vi "SR_J-Input Cycle.vi"(8 "error in (no error)":errorcluster, 10 "RDS Msg Q in":refnum<user-event>, 11 "Joystick":T1) -> (0 "error out":errorcluster, 2 "RDS Msg Q out":refnum<user-event>, 3 "Joystick Out":T1)   [LabVIEW 2015, in "Shore Library.lvlib"]
uses:
  Shore Library.lvlib
  SR-J-State.ctl
  Libraries/RDS Framework/RDS Message Class/RDS Message.lvclass
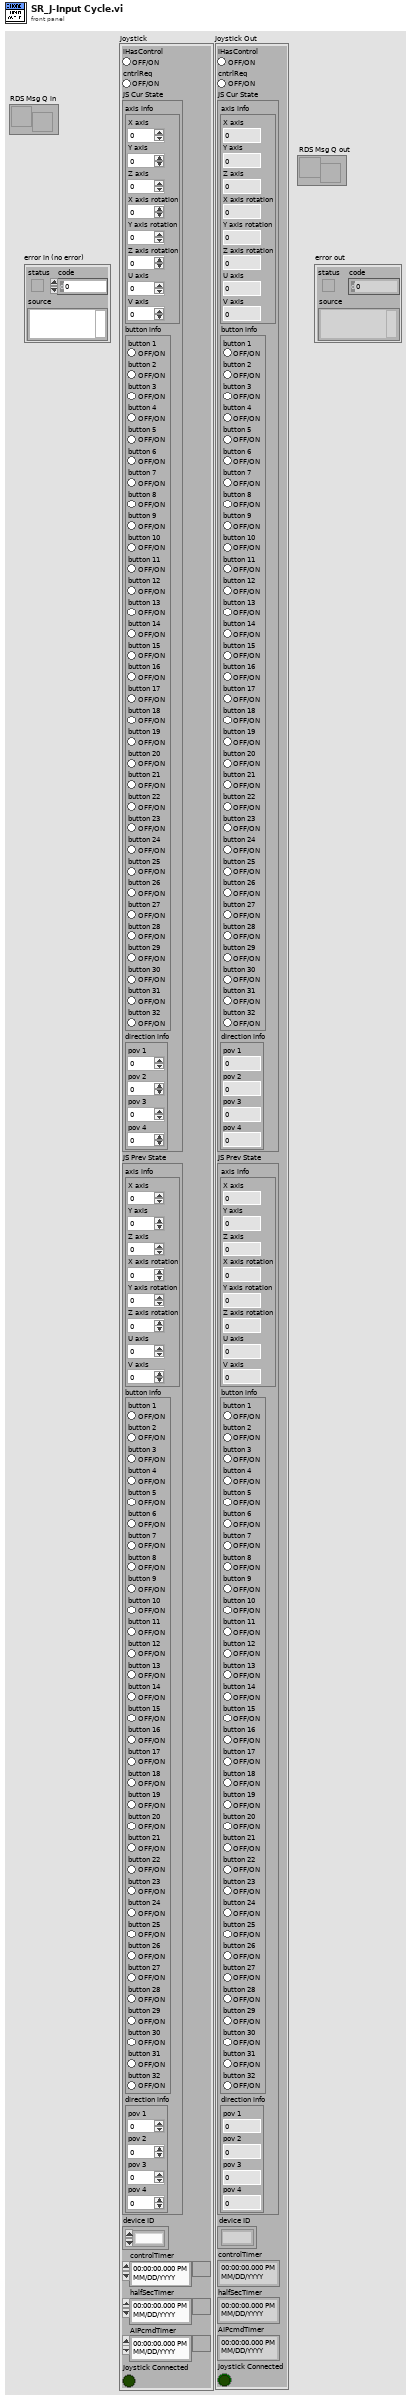
[diagram p1: front panel]
types:
  T1 = typedef "Shore Library.lvlib/SR-J-State.ctl" = cluster{"iHasControl":bool, "cntrlReq":bool, "JS Cur State":cluster{"axis info":cluster{"X axis":i32, "Y axis":i32, "Z axis":i32, "X axis rotation":i32, "Y axis rotation":i32, "Z axis rotation":i32, "U axis":i32, "V axis":i32}, "button info":cluster{"button 1":bool, "button 2":bool, "button 3":bool, "button 4":bool, "button 5":bool, "button 6":bool, "button 7":bool, "button 8":bool, "button 9":bool, "button 10":bool, "button 11":bool, "button 12":bool, "button 13":bool, "button 14":bool, "button 15":bool, "button 16":bool, "button 17":bool, "button 18":bool, "button 19":bool, "button 20":bool, "button 21":bool, "button 22":bool, "button 23":bool, "button 24":bool, "button 25":bool, "button 26":bool, "button 27":bool, "button 28":bool, "button 29":bool, "button 30":bool, "button 31":bool, "button 32":bool}, "direction info":cluster{"pov 1":i32, "pov 2":i32, "pov 3":i32, "pov 4":i32}}, "JS Prev State":cluster{"axis info":cluster{"X axis":i32, "Y axis":i32, "Z axis":i32, "X axis rotation":i32, "Y axis rotation":i32, "Z axis rotation":i32, "U axis":i32, "V axis":i32}, "button info":cluster{"button 1":bool, "button 2":bool, "button 3":bool, "button 4":bool, "button 5":bool, "button 6":bool, "button 7":bool, "button 8":bool, "button 9":bool, "button 10":bool, "button 11":bool, "button 12":bool, "button 13":bool, "button 14":bool, "button 15":bool, "button 16":bool, "button 17":bool, "button 18":bool, "button 19":bool, "button 20":bool, "button 21":bool, "button 22":bool, "button 23":bool, "button 24":bool, "button 25":bool, "button 26":bool, "button 27":bool, "button 28":bool, "button 29":bool, "button 30":bool, "button 31":bool, "button 32":bool}, "direction info":cluster{"pov 1":i32, "pov 2":i32, "pov 3":i32, "pov 4":i32}}, "device ID":refnum<k1>, "controlTimer":timestamp, "halfSecTimer":timestamp, "AIPcmdTimer":timestamp, "Joystick Connected":bool}
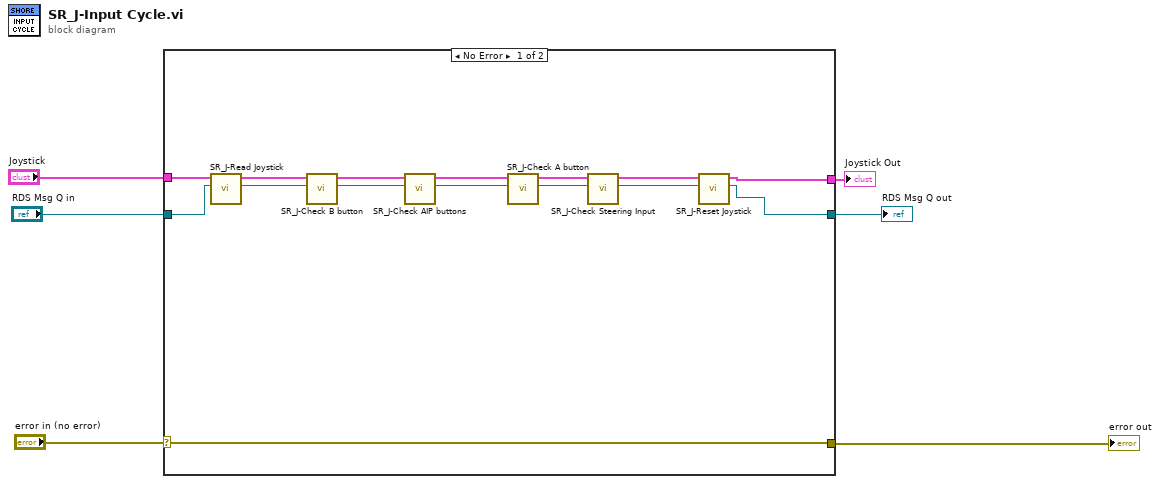
[diagram p0: block diagram]
diagram:
  n1 = case shown="No Error" "error in (no error)" {
    selector: "error in (no error)" -> [w21 w24]
    tunnel: [w21 w24] -> w5
    tunnel: "Joystick" -> [w10 w23]
    tunnel: "RDS Msg Q in" -> [w9 w22]
    tunnel: [w8 w23] -> w2
    tunnel: [w7 w22] -> w1
    frame No Error {
      n2 = call "SR_J-Read Joystick.vi"("RDS Msg Q in"=w9, "Joystick"=w10) -> ("RDS Msg Q out"=w15:refnum<user-event>, "Joystick Out"=w20:T1)  [unwired: 7 in, 1 out]
      n3 = call "SR_J-Check B button.vi"("RDS Message"=w15, "Joystick"=w20) -> ("RDS Message Out"=w14:refnum<user-event>, "Joystick out"=w19:T1)  [unwired: 7 in, 1 out]
      n4 = call "SR_J-Check AIP buttons.vi"("RDS Msg Q in"=w14, "Joystick"=w19) -> ("RDS Msg Q"=w13:refnum<user-event>, "Joystick Out"=w18:T1)  [unwired: 7 in, 1 out]
      n5 = call "SR_J-Check A button.vi"("RDS Msg Q in"=w13, "Joystick"=w18) -> ("RDS Msg Q out"=w12:refnum<user-event>, "Joystick 2"=w17:T1)  [unwired: 7 in, 1 out]
      n6 = call "SR_J-Check Steering Input.vi"("RDS Message"=w12, "Joystick"=w17) -> ("RDS Message out"=w11:refnum<user-event>, "Joystick 2"=w16:T1)  [unwired: 7 in, 1 out]
      n7 = call "SR_J-Reset Joystick.vi"("RDS Msg Q in"=w11, "Joystick in"=w16) -> ("RDS Msg Q out"=w7:refnum<user-event>, "Joystick Out"=w8:T1)  [unwired: 7 in, 1 out]
    }
    frame Error {
    }
  }
  "error out" <- w5
  "Joystick Out" <- w2
  "RDS Msg Q out" <- w1
